vi "Translate Coordinates.vi"(4 "Transformation Matrix":T1, 6 "Coordinates [pix]":cluster{"X":sgl, "Y":sgl}, 7 "FOV":cluster{"X [um]":dbl, "Y [um]":dbl} {"Y [um]" format="%.2f"; "X [um]" format="%.2f"}, 9 "Visualiser Zoom":cluster{"X":i32, "Y":i32}, 10 "Scope Position":T2, 11 "Image Area":cluster{"Width":u32, "Height":u32}) -> (1 "Target Coordinates":T2, 2 "coordinates [pix]":cluster{"X":sgl, "Y":sgl})   [LabVIEW 2012, in "Targeting Unit.lvlib"]
uses:
  Targeting Unit.lvlib
  <vilib>/Analysis/Matrix/Datatypes/RealMatrix.ctl
  <vilib>/Analysis/baseanly.llb/Real A x B.vi
  <vilib>/Analysis/NI_AALBase.lvlib
  <vilib>/Analysis/Matrix/NI_Matrix.lvlib
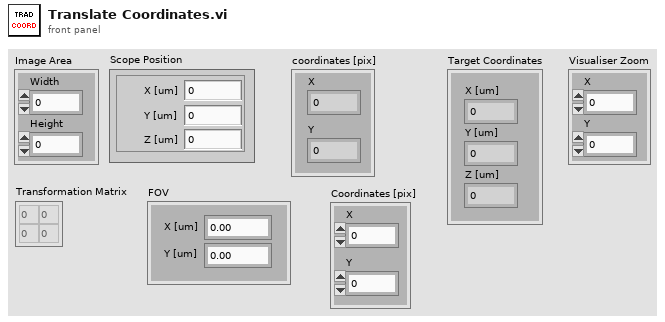
[diagram p1: front panel]
types:
  T1 = typedef "NI_Matrix.lvlib/RealMatrix.ctl" = dbl[][]
  T2 = cluster{"X [um]":dbl, "Y [um]":dbl, "Z [um]":dbl}
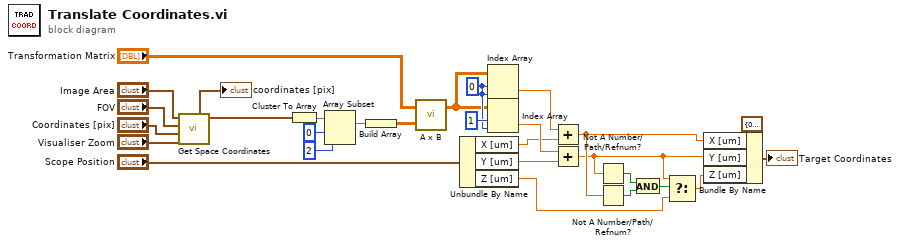
[diagram p0: block diagram]
diagram:
  w16 = 0 ("index (row)")
  n1 = call "Get Space Coordinates.vi"("Visualizer Zoom"="Visualiser Zoom", "coordinates [pix]"="Coordinates [pix]", "FOV"="FOV", "Image Area"="Image Area") -> ("coordinates [pix]"=→"coordinates [pix]":cluster{"X":sgl, "Y":sgl}, "coordinates [um]"=w14:cluster{"X [um]":dbl, "Y [um]":dbl})  [unwired: 6 in]
  n2 = Cluster To Array(cluster=w14) -> (array=w20:dbl[])
  n3 = Array Subset(array=w20, index=0, length=2) -> (w21:dbl[])
  n4 = Build Array(w21) -> (w23:T1)
  n5 = call-poly <vilib>:"A x B.vi"("B"=w23, "A"="Transformation Matrix") -> ("A x B"=w15:T1)  [unwired: 1 out]
  n6 = Unbundle By Name("Scope Position") -> ("X [um]"=w10:dbl, "Y [um]"=w13:dbl, "Z [um]"=w5:dbl)
  n7 = Index Array(array=w15, index (row)=w16, index (col)=w16) -> (element=w11:dbl)
  n8 = Index Array(array=w15, index (row)=1 ("index (col)"), index (col)=w16) -> (element=w12:dbl)
  n9 = Add ("Add.vi")(x=w11, y=w10) -> (x+y=w3:dbl)
  n10 = Add ("Add.vi")(x=w12, y=w13) -> (x+y=w2:dbl)
  n11 = Not A Number/Path/Refnum?(number/path/refnum=w2) -> (NaN/Path/Refnum?=w8:bool)
  n12 = Not A Number/Path/Refnum?(number/path/refnum=w3) -> (NaN/Path/Refnum?=w7:bool)
  n13 = And(x=w8, y=w7) -> (x .and. y?=w6:bool)
  n14 = Select(t=w2, s=w6, f=w5) -> (s? t:f=w4:dbl)
  n15 = Bundle By Name(cluster=T2 {"X [um]"=0.0, "Y [um]"=0.0, "Z [um]"=0.0} ("input cluster"), "X [um]"=w3, "Y [um]"=w2, "Z [um]"=w4) -> (→"Target Coordinates":T2)
